vi "main(Test DQMH modules).bak.vi"() -> ()   [LabVIEW 2018, in "Application.lvlib"] (continued)
          tunnel: w2879 -> [w2931]
          tunnel: w2872 -> [w2929]
          n1224 = Unbundle By Name(w2935) -> ("command"=w2934:string, "command data"=w2933:variant)
          n1225 = call "App enquece.vi"("Priority Enquece"=TRUE, "error in (no error)"=w2931, "command data"=w2933, "command"=w2934, "queue in"=w2929) -> ("error out"=w2932:errorcluster)  [unwired: 5 in, 1 out]
        }
        n1226 = Merge Errors(w2892, w2889) -> (w2893:errorcluster)
      }
      frame "Test Channel 8" {
        w2966 = 8  # DUT channel (1-11)
        w2967 = T11 {"command"="", "command data"=variant} ("element")
        n1227 = disable-structure shown="LOGGING==TRUE" {
          disable-tunnel: w2961 -> [w2996 _]
          frame condition #0 (active) {
            n1228 = Empty String/Path?(string/path=w2996) -> (empty?=w2999:bool)
            n1229 = Select(t="Quece timeout", s=w2999, f=w2996) -> (s? t:f=w2995:string)
            n1230 = call "string log (SubVI).vi"("Enum"=enum16{"Init", "Log", "Read"}."Log", "state Name"=w2995) -> ()  [unwired: 8 in, 2 out]
          }
          frame condition #1 {
          }
        }
        n1231 = Build Array("Apps.UI Update", "MEAS.AllRelaysOFF2", "Apps.WaitForEvent") -> (w2945:string[])
        n1232 = for {
          tunnel: [w2986] -> w2953 mode=indexing
          shift-right: [w2987] -> w2955
          shift-left: w2948 -> [w2985]
          tunnel: w2945 -> [w2984] mode=indexing
          n1233 = call "App enquece.vi"("Priority Enquece"=TRUE, "command"=w2984, "queue in"=w2985) -> ("error out"=w2986:errorcluster, "Queue out"=w2987:refnum<queue>)  [unwired: 7 in]
        }
        n1234 = Merge Errors(w2953) -> (w2944:errorcluster)
        n1235 = Build Array("Test DRV 43", "Test DRV 44", "Test DRV 45", "Test DRV 46", "Test DRV 47", "Test DRV 48", "MEAS.requestAC") -> (w2958:string[])
        n1236 = Reverse 1D Array(array=w2958) -> (reversed array=w2959:string[])
        n1237 = for {
          tunnel: w2959 -> [w2993] mode=indexing
          tunnel: [w2992] -> w2952 mode=indexing
          shift-right: [w2991] -> w2954
          shift-left: w2955 -> [w2994]
          tunnel: w2944 -> [w2990]
          n1238 = call "App enquece.vi"("Priority Enquece"=TRUE, "error in (no error)"=w2990, "command"=w2993, "queue in"=w2994) -> ("error out"=w2992:errorcluster, "Queue out"=w2991:refnum<queue>)  [unwired: 6 in]
        }
        n1239 = Initialize Array(TRUE, 6 ("dimension size")) -> (w2970:bool[])
        n1240 = Merge Errors(w2952) -> (w2951:errorcluster)
        n1241 = To Variant(anything=T5."mux10_1_channel8" ("mux10_1(x6)_encode")) -> (Variant=w2979:variant)
        n1242 = To Variant(anything=T6."demux1_10_channel8" ("demux1_10(x6)_encode")) -> (Variant=w2975:variant)
        n1243 = To Variant(anything=w2970) -> (Variant=w2969:variant)
        n1244 = Bundle By Name(cluster=w2967, "command"="MEAS.mux10-1", "command data"=w2979) -> (w2974:T11)
        n1245 = Bundle By Name(cluster=w2967, "command"="MEAS.demux1-10", "command data"=w2975) -> (w2973:T11)
        n1246 = Bundle By Name(cluster=w2967, "command"="MEAS.eMIC", "command data"=w2969) -> (w2968:T11)
        n1247 = Build Array(w2974, w2973, w2968) -> (w2950:T11[])
        n1248 = Reverse 1D Array(array=w2950) -> (reversed array=w2949:T11[])
        n1249 = for {
          tunnel: w2949 -> [w3005] mode=indexing
          tunnel: [w3002] -> w2960 mode=indexing
          tunnel: w2951 -> [w3001]
          tunnel: w2954 -> [w3006]
          n1250 = Unbundle By Name(w3005) -> ("command"=w3004:string, "command data"=w3003:variant)
          n1251 = call "App enquece.vi"("Priority Enquece"=TRUE, "error in (no error)"=w3001, "command data"=w3003, "command"=w3004, "queue in"=w3006) -> ("error out"=w3002:errorcluster)  [unwired: 5 in, 1 out]
        }
        n1252 = Merge Errors(w2963, w2960) -> (w2964:errorcluster)
      }
      frame "Test Channel 9" {
        w3038 = 9  # DUT channel (1-10)
        w3039 = T11 {"command"="", "command data"=variant} ("element")
        n1253 = disable-structure shown="LOGGING==TRUE" {
          disable-tunnel: w3033 -> [w3067 _]
          frame condition #0 (active) {
            n1254 = Empty String/Path?(string/path=w3067) -> (empty?=w3070:bool)
            n1255 = Select(t="Quece timeout", s=w3070, f=w3067) -> (s? t:f=w3066:string)
            n1256 = call "string log (SubVI).vi"("Enum"=enum16{"Init", "Log", "Read"}."Log", "state Name"=w3066) -> ()  [unwired: 8 in, 2 out]
          }
          frame condition #1 {
          }
        }
        n1257 = Build Array("Apps.UI Update", "MEAS.AllRelaysOFF2", "Apps.WaitForEvent") -> (w3015:string[])
        n1258 = for {
          tunnel: [w3057] -> w3024 mode=indexing
          shift-right: [w3058] -> w3026
          shift-left: w3019 -> [w3056]
          tunnel: w3015 -> [w3055] mode=indexing
          n1259 = call "App enquece.vi"("Priority Enquece"=TRUE, "command"=w3055, "queue in"=w3056) -> ("error out"=w3057:errorcluster, "Queue out"=w3058:refnum<queue>)  [unwired: 7 in]
        }
        n1260 = Merge Errors(w3024) -> (w3014:errorcluster)
        n1261 = Build Array("Test DRV 49", "Test DRV 50", "Test DRV 51", "Test DRV 52", "Test DRV 53", "Test DRV 54", "MEAS.requestAC") -> (w3030:string[])
        n1262 = Reverse 1D Array(array=w3030) -> (reversed array=w3031:string[])
        n1263 = for {
          tunnel: w3031 -> [w3064] mode=indexing
          tunnel: [w3063] -> w3023 mode=indexing
          shift-right: [w3062] -> w3025
          shift-left: w3026 -> [w3065]
          tunnel: w3014 -> [w3061]
          n1264 = call "App enquece.vi"("Priority Enquece"=TRUE, "error in (no error)"=w3061, "command"=w3064, "queue in"=w3065) -> ("error out"=w3063:errorcluster, "Queue out"=w3062:refnum<queue>)  [unwired: 6 in]
        }
        n1265 = Merge Errors(w3023) -> (w3022:errorcluster)
        n1266 = Initialize Array(TRUE, 6 ("dimension size")) -> (w3042:bool[])
        n1267 = To Variant(anything=T5."mux10_1_channel9" ("mux10_1(x6)_encode")) -> (Variant=w3051:variant)
        n1268 = To Variant(anything=T6."demux1_10_channel9" ("demux1_10(x6)_encode")) -> (Variant=w3047:variant)
        n1269 = To Variant(anything=w3042) -> (Variant=w3041:variant)
        n1270 = Bundle By Name(cluster=w3039, "command"="MEAS.mux10-1", "command data"=w3051) -> (w3046:T11)
        n1271 = Bundle By Name(cluster=w3039, "command"="MEAS.demux1-10", "command data"=w3047) -> (w3045:T11)
        n1272 = Bundle By Name(cluster=w3039, "command"="MEAS.eMIC", "command data"=w3041) -> (w3040:T11)
        n1273 = Build Array(w3046, w3045, w3040) -> (w3021:T11[])
        n1274 = Reverse 1D Array(array=w3021) -> (reversed array=w3020:T11[])
        n1275 = for {
          tunnel: w3020 -> [w3076] mode=indexing
          tunnel: [w3073] -> w3032 mode=indexing
          tunnel: w3022 -> [w3072]
          tunnel: w3025 -> [w3077]
          n1276 = Unbundle By Name(w3076) -> ("command"=w3075:string, "command data"=w3074:variant)
          n1277 = call "App enquece.vi"("Priority Enquece"=TRUE, "error in (no error)"=w3072, "command data"=w3074, "command"=w3075, "queue in"=w3077) -> ("error out"=w3073:errorcluster)  [unwired: 5 in, 1 out]
        }
        n1278 = Merge Errors(w3035, w3032) -> (w3036:errorcluster)
      }
      frame "Test Channel 10" {
        w3111 = 10  # DUT channel (1-10)
        w3087 = T11 {"command"="", "command data"=variant} ("element")
        n1279 = disable-structure shown="LOGGING==TRUE" {
          disable-tunnel: w3106 -> [w3138 _]
          frame condition #0 (active) {
            n1280 = Empty String/Path?(string/path=w3138) -> (empty?=w3141:bool)
            n1281 = Select(t="Quece timeout", s=w3141, f=w3138) -> (s? t:f=w3137:string)
            n1282 = call "string log (SubVI).vi"("Enum"=enum16{"Init", "Log", "Read"}."Log", "state Name"=w3137) -> ()  [unwired: 8 in, 2 out]
          }
          frame condition #1 {
          }
        }
        n1283 = Build Array("Apps.UI Update", "MEAS.AllRelaysOFF2", "Apps.WaitForEvent") -> (w3089:string[])
        n1284 = for {
          tunnel: [w3128] -> w3097 mode=indexing
          shift-right: [w3129] -> w3099
          shift-left: w3092 -> [w3127]
          tunnel: w3089 -> [w3126] mode=indexing
          n1285 = call "App enquece.vi"("Priority Enquece"=TRUE, "command"=w3126, "queue in"=w3127) -> ("error out"=w3128:errorcluster, "Queue out"=w3129:refnum<queue>)  [unwired: 7 in]
        }
        n1286 = Merge Errors(w3097) -> (w3088:errorcluster)
        n1287 = Build Array("Test DRV 55", "Test DRV 56", "Test DRV 57", "Test DRV 58", "Test DRV 59", "Test DRV 60", "MEAS.requestAC") -> (w3103:string[])
        n1288 = Reverse 1D Array(array=w3103) -> (reversed array=w3104:string[])
        n1289 = for {
          tunnel: w3104 -> [w3135] mode=indexing
          tunnel: [w3134] -> w3096 mode=indexing
          shift-right: [w3133] -> w3098
          shift-left: w3099 -> [w3136]
          tunnel: w3088 -> [w3132]
          n1290 = call "App enquece.vi"("Priority Enquece"=TRUE, "error in (no error)"=w3132, "command"=w3135, "queue in"=w3136) -> ("error out"=w3134:errorcluster, "Queue out"=w3133:refnum<queue>)  [unwired: 6 in]
        }
        n1291 = Initialize Array(TRUE, 6 ("dimension size")) -> (w3081:bool[])
        n1292 = To Variant(anything=T5."mux10_1_channel10" ("mux10_1(x6)_encode")) -> (Variant=w3121:variant)
        n1293 = To Variant(anything=T6."demux1_10_channel10" ("demux1_10(x6)_encode")) -> (Variant=w3117:variant)
        n1294 = To Variant(anything=w3081) -> (Variant=w3113:variant)
        n1295 = Bundle By Name(cluster=w3087, "command"="MEAS.mux10-1", "command data"=w3121) -> (w3116:T11)
        n1296 = Bundle By Name(cluster=w3087, "command"="MEAS.demux1-10", "command data"=w3117) -> (w3115:T11)
        n1297 = Bundle By Name(cluster=w3087, "command"="MEAS.eMIC", "command data"=w3113) -> (w3112:T11)
        n1298 = Merge Errors(w3096) -> (w3095:errorcluster)
        n1299 = Build Array(w3116, w3115, w3112) -> (w3094:T11[])
        n1300 = Reverse 1D Array(array=w3094) -> (reversed array=w3093:T11[])
        n1301 = for {
          tunnel: w3093 -> [w3147] mode=indexing
          tunnel: [w3144] -> w3105 mode=indexing
          tunnel: w3095 -> [w3143]
          tunnel: w3098 -> [w3148]
          n1302 = Unbundle By Name(w3147) -> ("command"=w3146:string, "command data"=w3145:variant)
          n1303 = call "App enquece.vi"("Priority Enquece"=TRUE, "error in (no error)"=w3143, "command data"=w3145, "command"=w3146, "queue in"=w3148) -> ("error out"=w3144:errorcluster)  [unwired: 5 in, 1 out]
        }
        n1304 = Merge Errors(w3108, w3105) -> (w3109:errorcluster)
      }
      frame "Test Channel 10A" {
        w3156 = T11 {"command"="", "command data"=variant} ("element")
        w3188 = 10  # DUT channel (1-10)
        w3167 = T11 {"command"="", "command data"=variant} ("element")
        n1305 = disable-structure shown="LOGGING==TRUE" {
          disable-tunnel: w3183 -> [w3217 _]
          frame condition #0 (active) {
            n1306 = Empty String/Path?(string/path=w3217) -> (empty?=w3220:bool)
            n1307 = Select(t="Quece timeout", s=w3220, f=w3217) -> (s? t:f=w3216:string)
            n1308 = call "string log (SubVI).vi"("Enum"=enum16{"Init", "Log", "Read"}."Log", "state Name"=w3216) -> ()  [unwired: 8 in, 2 out]
          }
          frame condition #1 {
          }
        }
        n1309 = Bundle By Name(cluster=w3156, "command"="Apps.UI Update", "command data"="A") -> (w3155:T11)
        n1310 = Bundle By Name(cluster=w3156, "command"="MEAS.AllRelaysOFF2") -> (w3154:T11)
        n1311 = Bundle By Name(cluster=w3156, "command"="Apps.WaitForEvent") -> (w3153:T11)
        n1312 = Build Array(w3155, w3154, w3153) -> (w3169:T11[])
        n1313 = for {
          tunnel: [w3207] -> w3176 mode=indexing
          shift-right: [w3208] -> w3178
          shift-left: w3171 -> [w3206]
          tunnel: w3169 -> [w3205] mode=indexing
          n1314 = Unbundle By Name(w3205) -> ("command"=w3204:string, "command data"=w3203:variant)
          n1315 = call "App enquece.vi"("Priority Enquece"=TRUE, "command data"=w3203, "command"=w3204, "queue in"=w3206) -> ("error out"=w3207:errorcluster, "Queue out"=w3208:refnum<queue>)  [unwired: 6 in]
        }
        n1316 = Merge Errors(w3176) -> (w3168:errorcluster)
        n1317 = Build Array("Test DRV 55", "Test DRV 56", "WaitFor", "MEAS.requestAC") -> (w3180:string[])
        n1318 = Reverse 1D Array(array=w3180) -> (reversed array=w3181:string[])
        n1319 = for {
          tunnel: w3181 -> [w3214] mode=indexing
          tunnel: [w3213] -> w3175 mode=indexing
          shift-right: [w3212] -> w3177
          shift-left: w3178 -> [w3215]
          tunnel: w3168 -> [w3211]
          n1320 = call "App enquece.vi"("Priority Enquece"=TRUE, "error in (no error)"=w3211, "command"=w3214, "queue in"=w3215) -> ("error out"=w3213:errorcluster, "Queue out"=w3212:refnum<queue>)  [unwired: 6 in]
        }
        n1321 = Initialize Array(TRUE, 2 ("dimension size")) -> (w3161:bool[])
        n1322 = Initialize Array(FALSE ("element"), 4 ("dimension size")) -> (w3160:bool[])
        n1323 = To Variant(anything=T5."mux10_1_channel10" ("mux10_1(x6)_encode")) -> (Variant=w3198:variant)
        n1324 = To Variant(anything=T6."demux1_10_channel10" ("demux1_10(x6)_encode")) -> (Variant=w3194:variant)
        n1325 = Build Array (concatenate)(w3161, w3160) -> (w3159:bool[])
        n1326 = To Variant(anything=w3159) -> (Variant=w3190:variant)
        n1327 = Bundle By Name(cluster=w3167, "command"="MEAS.mux10-1", "command data"=w3198) -> (w3193:T11)
        n1328 = Bundle By Name(cluster=w3167, "command"="MEAS.demux1-10", "command data"=w3194) -> (w3192:T11)
        n1329 = Bundle By Name(cluster=w3167, "command"="MEAS.eMIC", "command data"=w3190) -> (w3189:T11)
        n1330 = Merge Errors(w3175) -> (w3174:errorcluster)
        n1331 = Build Array(w3193, w3192, w3189) -> (w3173:T11[])
        n1332 = Reverse 1D Array(array=w3173) -> (reversed array=w3172:T11[])
        n1333 = for {
          tunnel: w3172 -> [w3226] mode=indexing
          tunnel: [w3223] -> w3182 mode=indexing
          tunnel: w3174 -> [w3222]
          tunnel: w3177 -> [w3227]
          n1334 = Unbundle By Name(w3226) -> ("command"=w3225:string, "command data"=w3224:variant)
          n1335 = call "App enquece.vi"("Priority Enquece"=TRUE, "error in (no error)"=w3222, "command data"=w3224, "command"=w3225, "queue in"=w3227) -> ("error out"=w3223:errorcluster)  [unwired: 5 in, 1 out]
        }
        n1336 = Merge Errors(w3185, w3182) -> (w3186:errorcluster)
      }
      frame "Test DRV 1" {
        w3229 = 1  # DUT index(1-60)
        n1337 = disable-structure shown="LOGGING==TRUE" {
          disable-tunnel: w3233 -> [w3266 _]
          frame condition #0 (active) {
            n1338 = Empty String/Path?(string/path=w3266) -> (empty?=w3269:bool)
            n1339 = Select(t="Quece timeout", s=w3269, f=w3266) -> (s? t:f=w3265:string)
            n1340 = call "string log (SubVI).vi"("Enum"=enum16{"Init", "Log", "Read"}."Log", "state Name"=w3265) -> ()  [unwired: 8 in, 2 out]
          }
          frame condition #1 {
          }
        }
        n1341 = call "progress string(SubVI).vi"("String 3"=w3233, "String in"=w3231) -> ("String out"=w3232:string)  [unwired: 9 in]
        n1342 = call "FGV Driver Data.vi"("DUT index(1-60)"=w3229, "FGV enum(Read)"=FGV_DRV_data."Read" ("FGV enum")) -> ("DUT SC"=w3230:bool)  [unwired: 6 in, 3 out]
        n1343 = case shown="False" w3230 {
          tunnel: [w3258 _] -> w3238
          tunnel: w3235 -> [w3257 _]
          frame False {
            w3245 = T11 {"command"="", "command data"=variant} ("element")
            w3244 = "MEAS.mux6_1"
            n1344 = To Variant(anything=T4."mux6_1_channel1_3" ("mux6_1(3wires)_encode")) -> (Variant=w3255:variant)
            n1345 = To Variant(anything=T4."mux6-1_channel0" ("mux6_1(3wires)_encode")) -> (Variant=w3243:variant)
            n1346 = To Variant(anything=T4."mux6-1_channel1_2" ("mux6_1(3wires)_encode")) -> (Variant=w3253:variant)
            n1347 = Bundle By Name(cluster=w3245, "command"=w3244, "command data"=w3253) -> (w3252:T11)
            n1348 = Bundle By Name(cluster=w3245, "command"=w3244, "command data"=w3255) -> (w3251:T11)
            n1349 = Bundle By Name(cluster=w3245, "command"=w3244, "command data"=w3243) -> ()  [unwired: 1 out]
            n1350 = Bundle By Name(cluster=w3245, "command"="MEAS.DMM dual read") -> (w3249:T11)
            n1351 = Build Array(w3252, w3251, w3249) -> (w3247:T11[])
            n1352 = Reverse 1D Array(array=w3247) -> (reversed array=w3248:T11[])
            n1353 = for {
              tunnel: [w3264] -> w3258 mode=indexing
              tunnel: w3257 -> [w3263]
              tunnel: w3248 -> [w3262] mode=indexing
              n1354 = Unbundle By Name(w3262) -> ("command"=w3261:string, "command data"=w3260:variant)
              n1355 = call "App enquece.vi"("Priority Enquece"=TRUE, "command data"=w3260, "command"=w3261, "queue in"=w3263) -> ("error out"=w3264:errorcluster)  [unwired: 6 in, 1 out]
            }
          }
          frame True {
          }
        }
        n1356 = Merge Errors(w3236, w3238) -> (w3237:errorcluster)
      }
      frame "Test DRV 2" {
        w3271 = 2  # DUT index(1-60)
        n1357 = disable-structure shown="LOGGING==TRUE" {
          disable-tunnel: w3272 -> [w3307 _]
          frame condition #0 (active) {
            n1358 = Empty String/Path?(string/path=w3307) -> (empty?=w3310:bool)
            n1359 = Select(t="Quece timeout", s=w3310, f=w3307) -> (s? t:f=w3306:string)
            n1360 = call "string log (SubVI).vi"("Enum"=enum16{"Init", "Log", "Read"}."Log", "state Name"=w3306) -> ()  [unwired: 8 in, 2 out]
          }
          frame condition #1 {
          }
        }
        n1361 = call "progress string(SubVI).vi"("String 3"=w3272, "String in"=w3273) -> ("String out"=w3274:string)  [unwired: 9 in]
        n1362 = call "FGV Driver Data.vi"("DUT index(1-60)"=w3271) -> ("DUT SC"=w3270:bool)  [unwired: 7 in, 3 out]
        n1363 = case shown="False" w3270 {
          tunnel: [w3299 _] -> w3279
          tunnel: w3276 -> [w3298 _]
          frame False {
            w3284 = T11 {"command"="", "command data"=variant} ("element")
            w3286 = "MEAS.mux6_1"
            n1364 = To Variant(anything=T4."mux6-1_channel0" ("mux6_1(3wires)_encode")) -> (Variant=w3285:variant)
            n1365 = To Variant(anything=T4."mux6_1_channel2_3" ("mux6_1(3wires)_encode")) -> (Variant=w3296:variant)
            n1366 = To Variant(anything=T4."mux6_1_channel2_2" ("mux6_1(3wires)_encode")) -> (Variant=w3294:variant)
            n1367 = Bundle By Name(cluster=w3284, "command"=w3286, "command data"=w3294) -> (w3293:T11)
            n1368 = Bundle By Name(cluster=w3284, "command"=w3286, "command data"=w3296) -> (w3292:T11)
            n1369 = Bundle By Name(cluster=w3284, "command"=w3286, "command data"=w3285) -> ()  [unwired: 1 out]
            n1370 = Bundle By Name(cluster=w3284, "command"="MEAS.DMM dual read") -> (w3290:T11)
            n1371 = Build Array(w3293, w3292, w3290) -> (w3288:T11[])
            n1372 = Reverse 1D Array(array=w3288) -> (reversed array=w3289:T11[])
            n1373 = for {
              tunnel: [w3305] -> w3299 mode=indexing
              tunnel: w3298 -> [w3304]
              tunnel: w3289 -> [w3303] mode=indexing
              n1374 = Unbundle By Name(w3303) -> ("command"=w3302:string, "command data"=w3301:variant)
              n1375 = call "App enquece.vi"("Priority Enquece"=TRUE, "command data"=w3301, "command"=w3302, "queue in"=w3304) -> ("error out"=w3305:errorcluster)  [unwired: 6 in, 1 out]
            }
          }
          frame True {
          }
        }
        n1376 = Merge Errors(w3277, w3279) -> (w3278:errorcluster)
      }
      frame "Test DRV 3" {
        w3312 = 3  # DUT index(1-60)
        n1377 = disable-structure shown="LOGGING==TRUE" {
          disable-tunnel: w3313 -> [w3348 _]
          frame condition #0 (active) {
            n1378 = Empty String/Path?(string/path=w3348) -> (empty?=w3351:bool)
            n1379 = Select(t="Quece timeout", s=w3351, f=w3348) -> (s? t:f=w3347:string)
            n1380 = call "string log (SubVI).vi"("Enum"=enum16{"Init", "Log", "Read"}."Log", "state Name"=w3347) -> ()  [unwired: 8 in, 2 out]
          }
          frame condition #1 {
          }
        }
        n1381 = call "progress string(SubVI).vi"("String 3"=w3313, "String in"=w3314) -> ("String out"=w3315:string)  [unwired: 9 in]
        n1382 = call "FGV Driver Data.vi"("DUT index(1-60)"=w3312) -> ("DUT SC"=w3311:bool)  [unwired: 7 in, 3 out]
        n1383 = case shown="False" w3311 {
          tunnel: [w3340 _] -> w3320
          tunnel: w3317 -> [w3339 _]
          frame False {
            w3327 = T11 {"command"="", "command data"=variant} ("element")
            w3326 = "MEAS.mux6_1"
            n1384 = To Variant(anything=T4."mux6-1_channel0" ("mux6_1(3wires)_encode")) -> (Variant=w3325:variant)
            n1385 = To Variant(anything=T4."mux6_1_channel3_3" ("mux6_1(3wires)_encode")) -> (Variant=w3337:variant)
            n1386 = To Variant(anything=T4."mux6_1_channel3_2" ("mux6_1(3wires)_encode")) -> (Variant=w3335:variant)
            n1387 = Bundle By Name(cluster=w3327, "command"=w3326, "command data"=w3335) -> (w3334:T11)
            n1388 = Bundle By Name(cluster=w3327, "command"=w3326, "command data"=w3337) -> (w3333:T11)
            n1389 = Bundle By Name(cluster=w3327, "command"=w3326, "command data"=w3325) -> ()  [unwired: 1 out]
            n1390 = Bundle By Name(cluster=w3327, "command"="MEAS.DMM dual read") -> (w3331:T11)
            n1391 = Build Array(w3334, w3333, w3331) -> (w3329:T11[])
            n1392 = Reverse 1D Array(array=w3329) -> (reversed array=w3330:T11[])
            n1393 = for {
              tunnel: [w3346] -> w3340 mode=indexing
              tunnel: w3339 -> [w3345]
              tunnel: w3330 -> [w3344] mode=indexing
              n1394 = Unbundle By Name(w3344) -> ("command"=w3343:string, "command data"=w3342:variant)
              n1395 = call "App enquece.vi"("Priority Enquece"=TRUE, "command data"=w3342, "command"=w3343, "queue in"=w3345) -> ("error out"=w3346:errorcluster)  [unwired: 6 in, 1 out]
            }
          }
          frame True {
          }
        }
        n1396 = Merge Errors(w3318, w3320) -> (w3319:errorcluster)
      }
      frame "Test DRV 4" {
        w3353 = 4  # DUT index(0-59)
        n1397 = disable-structure shown="LOGGING==TRUE" {
          disable-tunnel: w3354 -> [w3389 _]
          frame condition #0 (active) {
            n1398 = Empty String/Path?(string/path=w3389) -> (empty?=w3392:bool)
            n1399 = Select(t="Quece timeout", s=w3392, f=w3389) -> (s? t:f=w3388:string)
            n1400 = call "string log (SubVI).vi"("Enum"=enum16{"Init", "Log", "Read"}."Log", "state Name"=w3388) -> ()  [unwired: 8 in, 2 out]
          }
          frame condition #1 {
          }
        }
        n1401 = call "progress string(SubVI).vi"("String 3"=w3354, "String in"=w3355) -> ("String out"=w3356:string)  [unwired: 9 in]
        n1402 = call "FGV Driver Data.vi"("DUT index(1-60)"=w3353) -> ("DUT SC"=w3352:bool)  [unwired: 7 in, 3 out]
        n1403 = case shown="False" w3352 {
          tunnel: [w3381 _] -> w3361
          tunnel: w3358 -> [w3380 _]
          frame False {
            w3368 = T11 {"command"="", "command data"=variant} ("element")
            w3367 = "MEAS.mux6_1"
            n1404 = To Variant(anything=T4."mux6-1_channel0" ("mux6_1(3wires)_encode")) -> (Variant=w3366:variant)
            n1405 = To Variant(anything=T4."mux6_1_channel4_3" ("mux6_1(3wires)_encode")) -> (Variant=w3378:variant)
            n1406 = To Variant(anything=T4."mux6_1_channel4_2" ("mux6_1(3wires)_encode")) -> (Variant=w3376:variant)
            n1407 = Bundle By Name(cluster=w3368, "command"=w3367, "command data"=w3376) -> (w3375:T11)
            n1408 = Bundle By Name(cluster=w3368, "command"=w3367, "command data"=w3378) -> (w3374:T11)
            n1409 = Bundle By Name(cluster=w3368, "command"=w3367, "command data"=w3366) -> ()  [unwired: 1 out]
            n1410 = Bundle By Name(cluster=w3368, "command"="MEAS.DMM dual read") -> (w3372:T11)
            n1411 = Build Array(w3375, w3374, w3372) -> (w3370:T11[])
            n1412 = Reverse 1D Array(array=w3370) -> (reversed array=w3371:T11[])
            n1413 = for {
              tunnel: [w3387] -> w3381 mode=indexing
              tunnel: w3380 -> [w3386]
              tunnel: w3371 -> [w3385] mode=indexing
              n1414 = Unbundle By Name(w3385) -> ("command"=w3384:string, "command data"=w3383:variant)
              n1415 = call "App enquece.vi"("Priority Enquece"=TRUE, "command data"=w3383, "command"=w3384, "queue in"=w3386) -> ("error out"=w3387:errorcluster)  [unwired: 6 in, 1 out]
            }
          }
          frame True {
          }
        }
        n1416 = Merge Errors(w3359, w3361) -> (w3360:errorcluster)
      }
      frame "Test DRV 5" {
        w3394 = 5  # DUT index(0-59)
        n1417 = disable-structure shown="LOGGING==TRUE" {
          disable-tunnel: w3395 -> [w3430 _]
          frame condition #0 (active) {
            n1418 = Empty String/Path?(string/path=w3430) -> (empty?=w3433:bool)
            n1419 = Select(t="Quece timeout", s=w3433, f=w3430) -> (s? t:f=w3429:string)
            n1420 = call "string log (SubVI).vi"("Enum"=enum16{"Init", "Log", "Read"}."Log", "state Name"=w3429) -> ()  [unwired: 8 in, 2 out]
          }
          frame condition #1 {
          }
        }
        n1421 = call "progress string(SubVI).vi"("String 3"=w3395, "String in"=w3396) -> ("String out"=w3397:string)  [unwired: 9 in]
        n1422 = call "FGV Driver Data.vi"("DUT index(1-60)"=w3394) -> ("DUT SC"=w3393:bool)  [unwired: 7 in, 3 out]
        n1423 = case shown="False" w3393 {
          tunnel: [w3422 _] -> w3402
          tunnel: w3399 -> [w3421 _]
          frame False {
            w3409 = T11 {"command"="", "command data"=variant} ("element")
            w3408 = "MEAS.mux6_1"
            n1424 = To Variant(anything=T4."mux6-1_channel0" ("mux6_1(3wires)_encode")) -> (Variant=w3407:variant)
            n1425 = To Variant(anything=T4."mux6_1_channel5_3" ("mux6_1(3wires)_encode")) -> (Variant=w3419:variant)
            n1426 = To Variant(anything=T4."mux6_1_channel5_2" ("mux6_1(3wires)_encode")) -> (Variant=w3417:variant)
            n1427 = Bundle By Name(cluster=w3409, "command"=w3408, "command data"=w3417) -> (w3416:T11)
            n1428 = Bundle By Name(cluster=w3409, "command"=w3408, "command data"=w3419) -> (w3415:T11)
            n1429 = Bundle By Name(cluster=w3409, "command"=w3408, "command data"=w3407) -> ()  [unwired: 1 out]
            n1430 = Bundle By Name(cluster=w3409, "command"="MEAS.DMM dual read") -> (w3413:T11)
            n1431 = Build Array(w3416, w3415, w3413) -> (w3411:T11[])
            n1432 = Reverse 1D Array(array=w3411) -> (reversed array=w3412:T11[])
            n1433 = for {
              tunnel: [w3428] -> w3422 mode=indexing
              tunnel: w3421 -> [w3427]
              tunnel: w3412 -> [w3426] mode=indexing
              n1434 = Unbundle By Name(w3426) -> ("command"=w3425:string, "command data"=w3424:variant)
              n1435 = call "App enquece.vi"("Priority Enquece"=TRUE, "command data"=w3424, "command"=w3425, "queue in"=w3427) -> ("error out"=w3428:errorcluster)  [unwired: 6 in, 1 out]
            }
          }
          frame True {
          }
        }
        n1436 = Merge Errors(w3400, w3402) -> (w3401:errorcluster)
      }
      frame "Test DRV 6" {
        w3438 = 6  # DUT index(0-59)
        n1437 = disable-structure shown="LOGGING==TRUE" {
          disable-tunnel: w3434 -> [w3471 _]
          frame condition #0 (active) {
            n1438 = Empty String/Path?(string/path=w3471) -> (empty?=w3474:bool)
            n1439 = Select(t="Quece timeout", s=w3474, f=w3471) -> (s? t:f=w3470:string)
            n1440 = call "string log (SubVI).vi"("Enum"=enum16{"Init", "Log", "Read"}."Log", "state Name"=w3470) -> ()  [unwired: 8 in, 2 out]
          }
          frame condition #1 {
          }
        }
        n1441 = call "progress string(SubVI).vi"("String 3"=w3434, "String in"=w3435) -> ("String out"=w3436:string)  [unwired: 9 in]
        n1442 = call "FGV Driver Data.vi"("DUT index(1-60)"=w3438) -> ("DUT SC"=w3437:bool)  [unwired: 7 in, 3 out]
        n1443 = case shown="False" w3437 {
          tunnel: [w3463 _] -> w3443
          tunnel: w3440 -> [w3462 _]
          frame False {
            w3450 = T11 {"command"="", "command data"=variant} ("element")
            w3449 = "MEAS.mux6_1"
            n1444 = To Variant(anything=T4."mux6-1_channel0" ("mux6_1(3wires)_encode")) -> (Variant=w3448:variant)
            n1445 = To Variant(anything=T4."mux6_1_channel6_3" ("mux6_1(3wires)_encode")) -> (Variant=w3460:variant)
            n1446 = To Variant(anything=T4."mux6_1_channel6_2" ("mux6_1(3wires)_encode")) -> (Variant=w3458:variant)
            n1447 = Bundle By Name(cluster=w3450, "command"=w3449, "command data"=w3458) -> (w3457:T11)
            n1448 = Bundle By Name(cluster=w3450, "command"=w3449, "command data"=w3460) -> (w3456:T11)
            n1449 = Bundle By Name(cluster=w3450, "command"=w3449, "command data"=w3448) -> ()  [unwired: 1 out]
            n1450 = Bundle By Name(cluster=w3450, "command"="MEAS.DMM dual read") -> (w3454:T11)
            n1451 = Build Array(w3457, w3456, w3454) -> (w3452:T11[])
            n1452 = Reverse 1D Array(array=w3452) -> (reversed array=w3453:T11[])
            n1453 = for {
              tunnel: [w3469] -> w3463 mode=indexing
              tunnel: w3462 -> [w3468]
              tunnel: w3453 -> [w3467] mode=indexing
              n1454 = Unbundle By Name(w3467) -> ("command"=w3466:string, "command data"=w3465:variant)
              n1455 = call "App enquece.vi"("Priority Enquece"=TRUE, "command data"=w3465, "command"=w3466, "queue in"=w3468) -> ("error out"=w3469:errorcluster)  [unwired: 6 in, 1 out]
            }
          }
          frame True {
          }
        }
        n1456 = Merge Errors(w3441, w3443) -> (w3442:errorcluster)
      }
      frame "Test DRV 7" {
        w3476 = 7  # DUT index(0-59)
        n1457 = disable-structure shown="LOGGING==TRUE" {
          disable-tunnel: w3477 -> [w3512 _]
          frame condition #0 (active) {
            n1458 = Empty String/Path?(string/path=w3512) -> (empty?=w3515:bool)
            n1459 = Select(t="Quece timeout", s=w3515, f=w3512) -> (s? t:f=w3511:string)
            n1460 = call "string log (SubVI).vi"("Enum"=enum16{"Init", "Log", "Read"}."Log", "state Name"=w3511) -> ()  [unwired: 8 in, 2 out]
          }
          frame condition #1 {
          }
        }
        n1461 = call "progress string(SubVI).vi"("String 3"=w3477, "String in"=w3478) -> ("String out"=w3479:string)  [unwired: 9 in]
        n1462 = call "FGV Driver Data.vi"("DUT index(1-60)"=w3476) -> ("DUT SC"=w3475:bool)  [unwired: 7 in, 3 out]
        n1463 = case shown="False" w3475 {
          tunnel: [w3504 _] -> w3484
          tunnel: w3481 -> [w3503 _]
          frame False {
            w3491 = T11 {"command"="", "command data"=variant} ("element")
            w3490 = "MEAS.mux6_1"
            n1464 = To Variant(anything=T4."mux6-1_channel0" ("mux6_1(3wires)_encode")) -> (Variant=w3489:variant)
            n1465 = To Variant(anything=T4."mux6_1_channel1_3" ("mux6_1(3wires)_encode")) -> (Variant=w3501:variant)
            n1466 = To Variant(anything=T4."mux6-1_channel1_2" ("mux6_1(3wires)_encode")) -> (Variant=w3499:variant)
            n1467 = Bundle By Name(cluster=w3491, "command"=w3490, "command data"=w3499) -> (w3498:T11)
            n1468 = Bundle By Name(cluster=w3491, "command"=w3490, "command data"=w3501) -> (w3497:T11)
            n1469 = Bundle By Name(cluster=w3491, "command"=w3490, "command data"=w3489) -> ()  [unwired: 1 out]
            n1470 = Bundle By Name(cluster=w3491, "command"="MEAS.DMM dual read") -> (w3495:T11)
            n1471 = Build Array(w3498, w3497, w3495) -> (w3493:T11[])
            n1472 = Reverse 1D Array(array=w3493) -> (reversed array=w3494:T11[])
            n1473 = for {
              tunnel: [w3510] -> w3504 mode=indexing
              tunnel: w3503 -> [w3509]
              tunnel: w3494 -> [w3508] mode=indexing
              n1474 = Unbundle By Name(w3508) -> ("command"=w3507:string, "command data"=w3506:variant)
              n1475 = call "App enquece.vi"("Priority Enquece"=TRUE, "command data"=w3506, "command"=w3507, "queue in"=w3509) -> ("error out"=w3510:errorcluster)  [unwired: 6 in, 1 out]
            }
          }
          frame True {
          }
        }
        n1476 = Merge Errors(w3482, w3484) -> (w3483:errorcluster)
      }
      frame "Test DRV 8" {
        w3517 = 8  # DUT index(0-59)
        n1477 = disable-structure shown="LOGGING==TRUE" {
          disable-tunnel: w3518 -> [w3553 _]
          frame condition #0 (active) {
            n1478 = Empty String/Path?(string/path=w3553) -> (empty?=w3556:bool)
            n1479 = Select(t="Quece timeout", s=w3556, f=w3553) -> (s? t:f=w3552:string)
            n1480 = call "string log (SubVI).vi"("Enum"=enum16{"Init", "Log", "Read"}."Log", "state Name"=w3552) -> ()  [unwired: 8 in, 2 out]
          }
          frame condition #1 {
          }
        }
        n1481 = call "progress string(SubVI).vi"("String 3"=w3518, "String in"=w3519) -> ("String out"=w3520:string)  [unwired: 9 in]
        n1482 = call "FGV Driver Data.vi"("DUT index(1-60)"=w3517) -> ("DUT SC"=w3516:bool)  [unwired: 7 in, 3 out]
        n1483 = case shown="False" w3516 {
          tunnel: [w3545 _] -> w3525
          tunnel: w3522 -> [w3544 _]
          frame False {
            w3532 = T11 {"command"="", "command data"=variant} ("element")
            w3531 = "MEAS.mux6_1"
            n1484 = To Variant(anything=T4."mux6-1_channel0" ("mux6_1(3wires)_encode")) -> (Variant=w3530:variant)
            n1485 = To Variant(anything=T4."mux6_1_channel2_3" ("mux6_1(3wires)_encode")) -> (Variant=w3542:variant)
            n1486 = To Variant(anything=T4."mux6_1_channel2_2" ("mux6_1(3wires)_encode")) -> (Variant=w3540:variant)
            n1487 = Bundle By Name(cluster=w3532, "command"=w3531, "command data"=w3540) -> (w3539:T11)
            n1488 = Bundle By Name(cluster=w3532, "command"=w3531, "command data"=w3542) -> (w3538:T11)
            n1489 = Bundle By Name(cluster=w3532, "command"=w3531, "command data"=w3530) -> ()  [unwired: 1 out]
            n1490 = Bundle By Name(cluster=w3532, "command"="MEAS.DMM dual read") -> (w3536:T11)
            n1491 = Build Array(w3539, w3538, w3536) -> (w3534:T11[])
            n1492 = Reverse 1D Array(array=w3534) -> (reversed array=w3535:T11[])
            n1493 = for {
              tunnel: [w3551] -> w3545 mode=indexing
              tunnel: w3544 -> [w3550]
              tunnel: w3535 -> [w3549] mode=indexing
              n1494 = Unbundle By Name(w3549) -> ("command"=w3548:string, "command data"=w3547:variant)
              n1495 = call "App enquece.vi"("Priority Enquece"=TRUE, "command data"=w3547, "command"=w3548, "queue in"=w3550) -> ("error out"=w3551:errorcluster)  [unwired: 6 in, 1 out]
            }
          }
          frame True {
          }
        }
        n1496 = Merge Errors(w3523, w3525) -> (w3524:errorcluster)
      }
      frame "Test DRV 9" {
        w3558 = 9  # DUT index(0-59)
        n1497 = disable-structure shown="LOGGING==TRUE" {
          disable-tunnel: w3559 -> [w3594 _]
          frame condition #0 (active) {
            n1498 = Empty String/Path?(string/path=w3594) -> (empty?=w3597:bool)
            n1499 = Select(t="Quece timeout", s=w3597, f=w3594) -> (s? t:f=w3593:string)
            n1500 = call "string log (SubVI).vi"("Enum"=enum16{"Init", "Log", "Read"}."Log", "state Name"=w3593) -> ()  [unwired: 8 in, 2 out]
          }
          frame condition #1 {
          }
        }
        n1501 = call "progress string(SubVI).vi"("String 3"=w3559, "String in"=w3560) -> ("String out"=w3561:string)  [unwired: 9 in]
        n1502 = call "FGV Driver Data.vi"("DUT index(1-60)"=w3558) -> ("DUT SC"=w3557:bool)  [unwired: 7 in, 3 out]
        n1503 = case shown="False" w3557 {
          tunnel: [w3586 _] -> w3566
          tunnel: w3563 -> [w3585 _]
          frame False {
            w3573 = T11 {"command"="", "command data"=variant} ("element")
            w3572 = "MEAS.mux6_1"
            n1504 = To Variant(anything=T4."mux6-1_channel0" ("mux6_1(3wires)_encode")) -> (Variant=w3571:variant)
            n1505 = To Variant(anything=T4."mux6_1_channel3_3" ("mux6_1(3wires)_encode")) -> (Variant=w3583:variant)
            n1506 = To Variant(anything=T4."mux6_1_channel3_2" ("mux6_1(3wires)_encode")) -> (Variant=w3581:variant)
            n1507 = Bundle By Name(cluster=w3573, "command"=w3572, "command data"=w3581) -> (w3580:T11)
            n1508 = Bundle By Name(cluster=w3573, "command"=w3572, "command data"=w3583) -> (w3579:T11)
            n1509 = Bundle By Name(cluster=w3573, "command"=w3572, "command data"=w3571) -> ()  [unwired: 1 out]
            n1510 = Bundle By Name(cluster=w3573, "command"="MEAS.DMM dual read") -> (w3577:T11)
            n1511 = Build Array(w3580, w3579, w3577) -> (w3575:T11[])
            n1512 = Reverse 1D Array(array=w3575) -> (reversed array=w3576:T11[])
            n1513 = for {
              tunnel: [w3592] -> w3586 mode=indexing
              tunnel: w3585 -> [w3591]
              tunnel: w3576 -> [w3590] mode=indexing
              n1514 = Unbundle By Name(w3590) -> ("command"=w3589:string, "command data"=w3588:variant)
              n1515 = call "App enquece.vi"("Priority Enquece"=TRUE, "command data"=w3588, "command"=w3589, "queue in"=w3591) -> ("error out"=w3592:errorcluster)  [unwired: 6 in, 1 out]
            }
          }
          frame True {
          }
        }
        n1516 = Merge Errors(w3564, w3566) -> (w3565:errorcluster)
      }
      frame "Test DRV 10" {
        w3599 = 10  # DUT index(0-59)
        n1517 = disable-structure shown="LOGGING==TRUE" {
          disable-tunnel: w3600 -> [w3635 _]
          frame condition #0 (active) {
            n1518 = Empty String/Path?(string/path=w3635) -> (empty?=w3638:bool)
            n1519 = Select(t="Quece timeout", s=w3638, f=w3635) -> (s? t:f=w3634:string)
            n1520 = call "string log (SubVI).vi"("Enum"=enum16{"Init", "Log", "Read"}."Log", "state Name"=w3634) -> ()  [unwired: 8 in, 2 out]
          }
          frame condition #1 {
          }
        }
        n1521 = call "progress string(SubVI).vi"("String 3"=w3600, "String in"=w3601) -> ("String out"=w3602:string)  [unwired: 9 in]
        n1522 = call "FGV Driver Data.vi"("DUT index(1-60)"=w3599) -> ("DUT SC"=w3598:bool)  [unwired: 7 in, 3 out]
        n1523 = case shown="False" w3598 {
          tunnel: [w3627 _] -> w3607
          tunnel: w3604 -> [w3626 _]
          frame False {
            w3614 = T11 {"command"="", "command data"=variant} ("element")
            w3613 = "MEAS.mux6_1"
            n1524 = To Variant(anything=T4."mux6-1_channel0" ("mux6_1(3wires)_encode")) -> (Variant=w3612:variant)
            n1525 = To Variant(anything=T4."mux6_1_channel4_3" ("mux6_1(3wires)_encode")) -> (Variant=w3624:variant)
            n1526 = To Variant(anything=T4."mux6_1_channel4_2" ("mux6_1(3wires)_encode")) -> (Variant=w3622:variant)
            n1527 = Bundle By Name(cluster=w3614, "command"=w3613, "command data"=w3622) -> (w3621:T11)
            n1528 = Bundle By Name(cluster=w3614, "command"=w3613, "command data"=w3624) -> (w3620:T11)
            n1529 = Bundle By Name(cluster=w3614, "command"=w3613, "command data"=w3612) -> ()  [unwired: 1 out]
            n1530 = Bundle By Name(cluster=w3614, "command"="MEAS.DMM dual read") -> (w3618:T11)
            n1531 = Build Array(w3621, w3620, w3618) -> (w3616:T11[])
            n1532 = Reverse 1D Array(array=w3616) -> (reversed array=w3617:T11[])
            n1533 = for {
              tunnel: [w3633] -> w3627 mode=indexing
              tunnel: w3626 -> [w3632]
              tunnel: w3617 -> [w3631] mode=indexing
              n1534 = Unbundle By Name(w3631) -> ("command"=w3630:string, "command data"=w3629:variant)
              n1535 = call "App enquece.vi"("Priority Enquece"=TRUE, "command data"=w3629, "command"=w3630, "queue in"=w3632) -> ("error out"=w3633:errorcluster)  [unwired: 6 in, 1 out]
            }
          }
          frame True {
          }
        }
        n1536 = Merge Errors(w3605, w3607) -> (w3606:errorcluster)
      }
      frame "Test DRV 11" {
        w3640 = 11  # DUT index(0-59)
        n1537 = disable-structure shown="LOGGING==TRUE" {
          disable-tunnel: w3641 -> [w3676 _]
          frame condition #0 (active) {
            n1538 = Empty String/Path?(string/path=w3676) -> (empty?=w3679:bool)
            n1539 = Select(t="Quece timeout", s=w3679, f=w3676) -> (s? t:f=w3675:string)
            n1540 = call "string log (SubVI).vi"("Enum"=enum16{"Init", "Log", "Read"}."Log", "state Name"=w3675) -> ()  [unwired: 8 in, 2 out]
          }
          frame condition #1 {
          }
        }
        n1541 = call "progress string(SubVI).vi"("String 3"=w3641, "String in"=w3642) -> ("String out"=w3643:string)  [unwired: 9 in]
        n1542 = call "FGV Driver Data.vi"("DUT index(1-60)"=w3640) -> ("DUT SC"=w3639:bool)  [unwired: 7 in, 3 out]
        n1543 = case shown="False" w3639 {
          tunnel: [w3668 _] -> w3648
          tunnel: w3645 -> [w3667 _]
          frame False {
            w3653 = T11 {"command"="", "command data"=variant} ("element")
            w3655 = "MEAS.mux6_1"
            n1544 = To Variant(anything=T4."mux6-1_channel0" ("mux6_1(3wires)_encode")) -> (Variant=w3654:variant)
            n1545 = To Variant(anything=T4."mux6_1_channel5_3" ("mux6_1(3wires)_encode")) -> (Variant=w3665:variant)
            n1546 = To Variant(anything=T4."mux6_1_channel5_2" ("mux6_1(3wires)_encode")) -> (Variant=w3663:variant)
            n1547 = Bundle By Name(cluster=w3653, "command"=w3655, "command data"=w3663) -> (w3662:T11)
            n1548 = Bundle By Name(cluster=w3653, "command"=w3655, "command data"=w3665) -> (w3661:T11)
            n1549 = Bundle By Name(cluster=w3653, "command"=w3655, "command data"=w3654) -> ()  [unwired: 1 out]
            n1550 = Bundle By Name(cluster=w3653, "command"="MEAS.DMM dual read") -> (w3659:T11)
            n1551 = Build Array(w3662, w3661, w3659) -> (w3657:T11[])
            n1552 = Reverse 1D Array(array=w3657) -> (reversed array=w3658:T11[])
            n1553 = for {
              tunnel: [w3674] -> w3668 mode=indexing
              tunnel: w3667 -> [w3673]
              tunnel: w3658 -> [w3672] mode=indexing
              n1554 = Unbundle By Name(w3672) -> ("command"=w3671:string, "command data"=w3670:variant)
              n1555 = call "App enquece.vi"("Priority Enquece"=TRUE, "command data"=w3670, "command"=w3671, "queue in"=w3673) -> ("error out"=w3674:errorcluster)  [unwired: 6 in, 1 out]
            }
          }
          frame True {
          }
        }
        n1556 = Merge Errors(w3646, w3648) -> (w3647:errorcluster)
      }
      frame "Test DRV 12" {
        w3681 = 12  # DUT index(0-59)
        n1557 = disable-structure shown="LOGGING==TRUE" {
          disable-tunnel: w3682 -> [w3717 _]
          frame condition #0 (active) {
            n1558 = Empty String/Path?(string/path=w3717) -> (empty?=w3720:bool)
            n1559 = Select(t="Quece timeout", s=w3720, f=w3717) -> (s? t:f=w3716:string)
            n1560 = call "string log (SubVI).vi"("Enum"=enum16{"Init", "Log", "Read"}."Log", "state Name"=w3716) -> ()  [unwired: 8 in, 2 out]
          }
          frame condition #1 {
          }
        }
        n1561 = call "progress string(SubVI).vi"("String 3"=w3682, "String in"=w3683) -> ("String out"=w3684:string)  [unwired: 9 in]
        n1562 = call "FGV Driver Data.vi"("DUT index(1-60)"=w3681) -> ("DUT SC"=w3680:bool)  [unwired: 7 in, 3 out]
        n1563 = case shown="False" w3680 {
          tunnel: [w3709 _] -> w3689
          tunnel: w3686 -> [w3708 _]
          frame False {
            w3696 = T11 {"command"="", "command data"=variant} ("element")
            w3695 = "MEAS.mux6_1"
            n1564 = To Variant(anything=T4."mux6-1_channel0" ("mux6_1(3wires)_encode")) -> (Variant=w3694:variant)
            n1565 = To Variant(anything=T4."mux6_1_channel6_3" ("mux6_1(3wires)_encode")) -> (Variant=w3706:variant)
            n1566 = To Variant(anything=T4."mux6_1_channel6_2" ("mux6_1(3wires)_encode")) -> (Variant=w3704:variant)
            n1567 = Bundle By Name(cluster=w3696, "command"=w3695, "command data"=w3704) -> (w3703:T11)
            n1568 = Bundle By Name(cluster=w3696, "command"=w3695, "command data"=w3706) -> (w3702:T11)
            n1569 = Bundle By Name(cluster=w3696, "command"=w3695, "command data"=w3694) -> ()  [unwired: 1 out]
            n1570 = Bundle By Name(cluster=w3696, "command"="MEAS.DMM dual read") -> (w3700:T11)
            n1571 = Build Array(w3703, w3702, w3700) -> (w3698:T11[])
            n1572 = Reverse 1D Array(array=w3698) -> (reversed array=w3699:T11[])
            n1573 = for {
              tunnel: [w3715] -> w3709 mode=indexing
              tunnel: w3708 -> [w3714]
              tunnel: w3699 -> [w3713] mode=indexing
              n1574 = Unbundle By Name(w3713) -> ("command"=w3712:string, "command data"=w3711:variant)
              n1575 = call "App enquece.vi"("Priority Enquece"=TRUE, "command data"=w3711, "command"=w3712, "queue in"=w3714) -> ("error out"=w3715:errorcluster)  [unwired: 6 in, 1 out]
            }
          }
          frame True {
          }
        }
        n1576 = Merge Errors(w3687, w3689) -> (w3688:errorcluster)
      }
      frame "Test DRV 13" {
        w3722 = 13  # DUT index(0-59)
        n1577 = disable-structure shown="LOGGING==TRUE" {
          disable-tunnel: w3723 -> [w3758 _]
          frame condition #0 (active) {
            n1578 = Empty String/Path?(string/path=w3758) -> (empty?=w3761:bool)
            n1579 = Select(t="Quece timeout", s=w3761, f=w3758) -> (s? t:f=w3757:string)
            n1580 = call "string log (SubVI).vi"("Enum"=enum16{"Init", "Log", "Read"}."Log", "state Name"=w3757) -> ()  [unwired: 8 in, 2 out]
          }
          frame condition #1 {
          }
        }
        n1581 = call "progress string(SubVI).vi"("String 3"=w3723, "String in"=w3724) -> ("String out"=w3725:string)  [unwired: 9 in]
        n1582 = call "FGV Driver Data.vi"("DUT index(1-60)"=w3722) -> ("DUT SC"=w3721:bool)  [unwired: 7 in, 3 out]
        n1583 = case shown="False" w3721 {
          tunnel: [w3750 _] -> w3730
          tunnel: w3727 -> [w3749 _]
          frame False {
            w3737 = T11 {"command"="", "command data"=variant} ("element")
            w3736 = "MEAS.mux6_1"
            n1584 = To Variant(anything=T4."mux6-1_channel0" ("mux6_1(3wires)_encode")) -> (Variant=w3735:variant)
            n1585 = To Variant(anything=T4."mux6_1_channel1_3" ("mux6_1(3wires)_encode")) -> (Variant=w3747:variant)
            n1586 = To Variant(anything=T4."mux6-1_channel1_2" ("mux6_1(3wires)_encode")) -> (Variant=w3745:variant)
            n1587 = Bundle By Name(cluster=w3737, "command"=w3736, "command data"=w3745) -> (w3744:T11)
            n1588 = Bundle By Name(cluster=w3737, "command"=w3736, "command data"=w3747) -> (w3743:T11)
            n1589 = Bundle By Name(cluster=w3737, "command"=w3736, "command data"=w3735) -> ()  [unwired: 1 out]
            n1590 = Bundle By Name(cluster=w3737, "command"="MEAS.DMM dual read") -> (w3741:T11)
            n1591 = Build Array(w3744, w3743, w3741) -> (w3739:T11[])
            n1592 = Reverse 1D Array(array=w3739) -> (reversed array=w3740:T11[])
            n1593 = for {
              tunnel: [w3756] -> w3750 mode=indexing
              tunnel: w3749 -> [w3755]
              tunnel: w3740 -> [w3754] mode=indexing
              n1594 = Unbundle By Name(w3754) -> ("command"=w3753:string, "command data"=w3752:variant)
              n1595 = call "App enquece.vi"("Priority Enquece"=TRUE, "command data"=w3752, "command"=w3753, "queue in"=w3755) -> ("error out"=w3756:errorcluster)  [unwired: 6 in, 1 out]
            }
          }
          frame True {
          }
        }
        n1596 = Merge Errors(w3728, w3730) -> (w3729:errorcluster)
      }
      frame "Test DRV 14" {
        w3763 = 14  # DUT index(0-59)
        n1597 = disable-structure shown="LOGGING==TRUE" {
          disable-tunnel: w3764 -> [w3799 _]
          frame condition #0 (active) {
            n1598 = Empty String/Path?(string/path=w3799) -> (empty?=w3802:bool)
            n1599 = Select(t="Quece timeout", s=w3802, f=w3799) -> (s? t:f=w3798:string)
            n1600 = call "string log (SubVI).vi"("Enum"=enum16{"Init", "Log", "Read"}."Log", "state Name"=w3798) -> ()  [unwired: 8 in, 2 out]
          }
          frame condition #1 {
          }
        }
        n1601 = call "progress string(SubVI).vi"("String 3"=w3764, "String in"=w3765) -> ("String out"=w3766:string)  [unwired: 9 in]
        n1602 = call "FGV Driver Data.vi"("DUT index(1-60)"=w3763) -> ("DUT SC"=w3762:bool)  [unwired: 7 in, 3 out]
        n1603 = case shown="False" w3762 {
          tunnel: [w3791 _] -> w3771
          tunnel: w3768 -> [w3790 _]
          frame False {
            w3778 = T11 {"command"="", "command data"=variant} ("element")
            w3777 = "MEAS.mux6_1"
            n1604 = To Variant(anything=T4."mux6_1_channel2_3" ("mux6_1(3wires)_encode")) -> (Variant=w3788:variant)
            n1605 = To Variant(anything=T4."mux6-1_channel0" ("mux6_1(3wires)_encode")) -> (Variant=w3776:variant)
            n1606 = To Variant(anything=T4."mux6_1_channel2_2" ("mux6_1(3wires)_encode")) -> (Variant=w3786:variant)
            n1607 = Bundle By Name(cluster=w3778, "command"=w3777, "command data"=w3786) -> (w3785:T11)
            n1608 = Bundle By Name(cluster=w3778, "command"=w3777, "command data"=w3788) -> (w3784:T11)
            n1609 = Bundle By Name(cluster=w3778, "command"=w3777, "command data"=w3776) -> ()  [unwired: 1 out]
            n1610 = Bundle By Name(cluster=w3778, "command"="MEAS.DMM dual read") -> (w3782:T11)
            n1611 = Build Array(w3785, w3784, w3782) -> (w3780:T11[])
            n1612 = Reverse 1D Array(array=w3780) -> (reversed array=w3781:T11[])
            n1613 = for {
              tunnel: [w3797] -> w3791 mode=indexing
              tunnel: w3790 -> [w3796]
              tunnel: w3781 -> [w3795] mode=indexing
              n1614 = Unbundle By Name(w3795) -> ("command"=w3794:string, "command data"=w3793:variant)
              n1615 = call "App enquece.vi"("Priority Enquece"=TRUE, "command data"=w3793, "command"=w3794, "queue in"=w3796) -> ("error out"=w3797:errorcluster)  [unwired: 6 in, 1 out]
            }
          }
          frame True {
          }
        }
        n1616 = Merge Errors(w3769, w3771) -> (w3770:errorcluster)
      }
      frame "Test DRV 15" {
        w3804 = 15  # DUT index(0-59)
        n1617 = disable-structure shown="LOGGING==TRUE" {
          disable-tunnel: w3805 -> [w3840 _]
          frame condition #0 (active) {
            n1618 = Empty String/Path?(string/path=w3840) -> (empty?=w3843:bool)
            n1619 = Select(t="Quece timeout", s=w3843, f=w3840) -> (s? t:f=w3839:string)
            n1620 = call "string log (SubVI).vi"("Enum"=enum16{"Init", "Log", "Read"}."Log", "state Name"=w3839) -> ()  [unwired: 8 in, 2 out]
          }
          frame condition #1 {
          }
        }
